vi "Create Test Designs.vi"(6 "Config":T1=enum."Write", 8 "error in (no error)":errorcluster, 9 "Method Index":i32, 10 "Methods":string[](array[string])=["EtFlocSedFiLow", "EtFlocSedFi", "Flocculator", "SedTank", "SRSF", "LFOM", "Cdc", "Box"], 11 "ADT version":i32) -> (0 "error out":errorcluster)   [LabVIEW 2011]
uses:
  ReadWrite.ctl
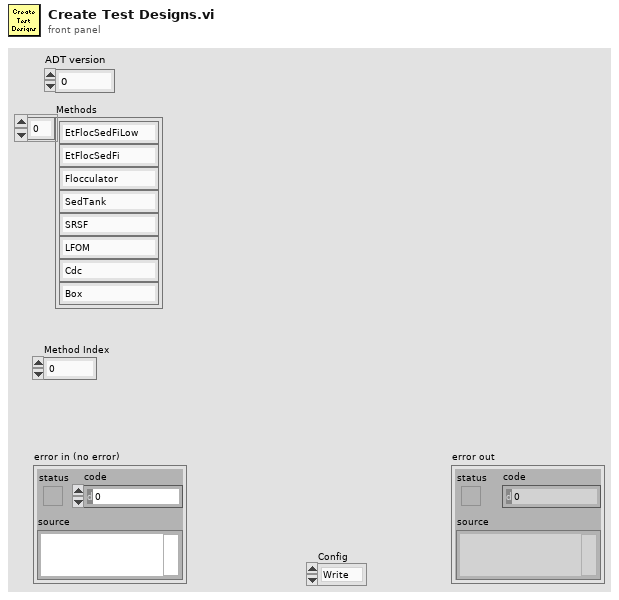
[diagram p1: front panel]
types:
  T1 = typedef "ReadWrite.ctl" = enum16{"Read", "Write"}
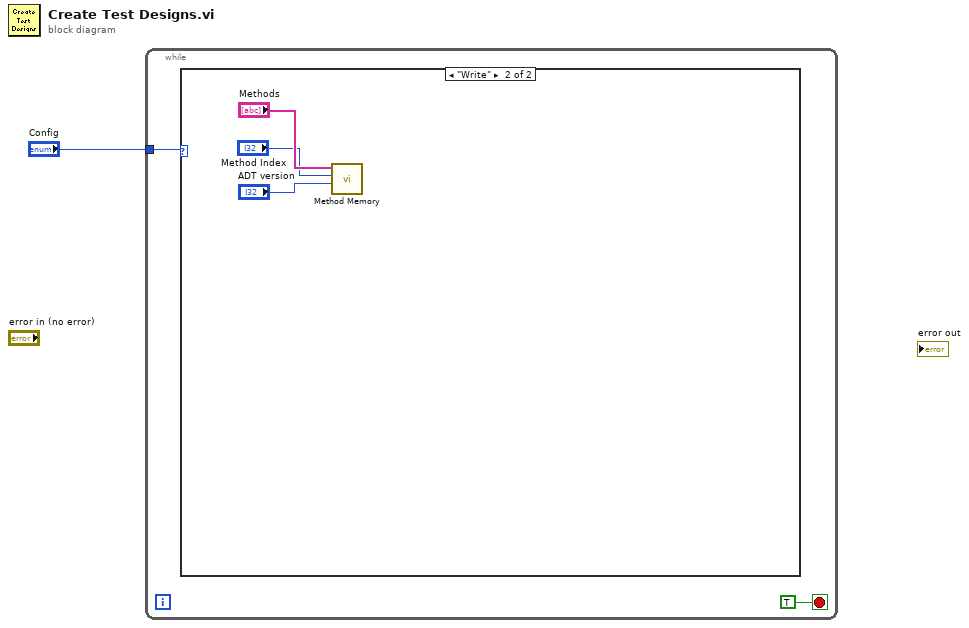
[diagram p0: block diagram]
diagram:
  n1 = while {
    tunnel: "Config" -> [w2]
    stop <- TRUE stop-if-true
    n2 = case shown="\"Write\"" w2 {
      frame "Read", Default {
      }
      frame "Write" {
        n3 = call "Method Memory.vi"(9:"ADT version", "ADT version"="Method Index", "Method Name"="Methods") -> ()  [unwired: 6 in, 3 out]
      }
    }
  }
